vi "SinglePinSingleSiteReservation_CallGetConnectionFromPin_ReturnsSingleConnection.vi"(8 "error in":errorcluster) -> (0 "error out":errorcluster, 2 "result":string, 3 "pass":bool)   [LabVIEW 2020, in "MeasurementServerTests.lvlib"]
uses:
  MeasurementServerTests.lvlib
  Runtime/MeasurementLink Session Management/Session Reservation/Connection.ctl
  Runtime/MeasurementLink Session Management/Session Reservation/Hardware Independent Connection.ctl
  8c161b2c-7580-4f71-9eec-17cc94e5f6f8.vi
  b3e5c3be-b7a7-4b6e-86ee-709eea9cb752.vi
  8c161b2c-7580-4f71-9eec-17cc94e5f6f8.vi/d089b476-b30c-4b91-b2ff-fbae0086b065.vi
  Runtime/MeasurementLink Session Management/Session Reservation/Get Connections Impl.vi
  <vilib>/Utility/error.llb/Error Cluster From Error Code.vi
  Runtime/MeasurementLink Session Management/Session Reservation/Session Reservation.lvclass
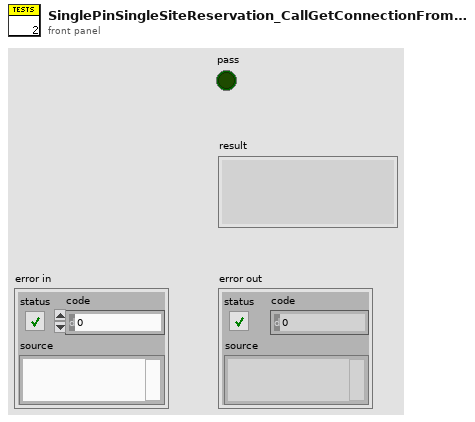
[diagram p1: front panel]
types:
  T1 = typedef "MeasurementLink Session Management.lvlib/Session Reservation.lvclass/Connection.ctl" = cluster{"connection":T2, "session":variant}
  T2 = typedef "MeasurementLink Session Management.lvlib/Session Reservation.lvclass/Hardware Independent Connection.ctl" = cluster{"pin or relay name":string, "site":i32, "instrument type id":string, "channel":string}
  T3 = typedef "MeasurementLink Session Management Client.lvlib/ni_measurementlink_sessionmanagement_v1_ChannelMapping.ctl" = cluster{"pin_or_relay_name":string, "site":i32, "channel":string}
  T4 = typedef "MeasurementLink Session Management.lvlib/Session Reservation.lvclass/Data.ctl" = cluster{"session and driver infos":T5[], "pins":string[]}
  T5 = typedef "MeasurementLink Session Management.lvlib/Session Reservation.lvclass/Session and Driver Info.ctl" = cluster{"session info":T6, "session created":bool, "session":variant}
  T6 = typedef "MeasurementLink Session Management Client.lvlib/ni_measurementlink_sessionmanagement_v1_SessionInformation.ctl" = cluster{"session":T7, "resource_name":string, "channel_list":string, "instrument_type_id":string, "session_exists":bool, "channel_mappings":T3[]}
  T7 = typedef "MeasurementLink Session Management Client.lvlib/nidevice_grpc_Session.ctl" = cluster{"name":string}
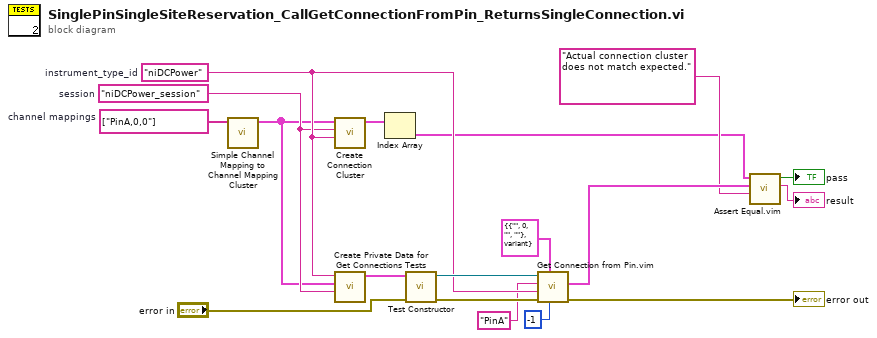
[diagram p0: block diagram]
diagram:
  w5 = string[] ["PinA,0,0"]  # channel mappings
  w10 = "niDCPower_session"  # session
  w11 = "niDCPower"  # instrument_type_id
  n1 = call "Simple Channel Mapping to Channel Mapping Cluster.vi"("simple channel mappings"=w5) -> ("channel mappings"=w3:T3[])  [unwired: 10 in]
  n2 = call "Create Connection Cluster.vi"("instrument_type_id"=w11, "session"=w10, "channel mappings"=w3) -> ("connections"=w1:T1[])  [unwired: 8 in]
  n3 = call "Create Private Data for Get Connections Tests.vi"("session"=w10, "channel mappings"=w3, "instrument_type_id"=w11) -> ("data"=w12:T4)  [unwired: 8 in]
  n4 = Index Array(array=w1) -> (element=w2:T1)  [unwired: 1 in]
  n5 = call "Test Constructor.vi"("error in"="error in", "data"=w12) -> ("error out"=w17:errorcluster, "Session Reservation out"=w16:refnum<class "Session Reservation.lvclass">)  [unwired: 8 in]
  n6 = call "Get Connection from Pin.vim"("site"=-1, "connection type"=T1 {"connection"={"pin or relay name"="", "site"=0, "instrument type id"="", "channel"=""}, "session"=variant} ("connection"), "error in"=w17, "instrument type id"=w11, "pin or relay name"="PinA", "session reservation in"=w16) -> ("error out"=→"error out":errorcluster, "connection"=w9:T1)  [unwired: 3 in, 1 out]
  n7 = call "Assert Equal.vim"("failure message"="Actual connection cluster does not match expected.", "actual value"=w9, "expected value"=w2) -> ("message"=→"result":string, "equal?"=→"pass":bool)  [unwired: 7 in]
